vi "instance count allowed.vi"(8 "error in":errorcluster, 11 "WaveformAcq configuration in":refnum<class "WaveformAcq configuration.lvclass">) -> (0 "error out":errorcluster, 2 "instances allowed":i32, 3 "WaveformAcq configuration out":refnum<class "WaveformAcq configuration.lvclass">)   [LabVIEW 2017, in "WaveformAcq configuration.lvclass"]
uses:
  WaveformAcq configuration.lvclass
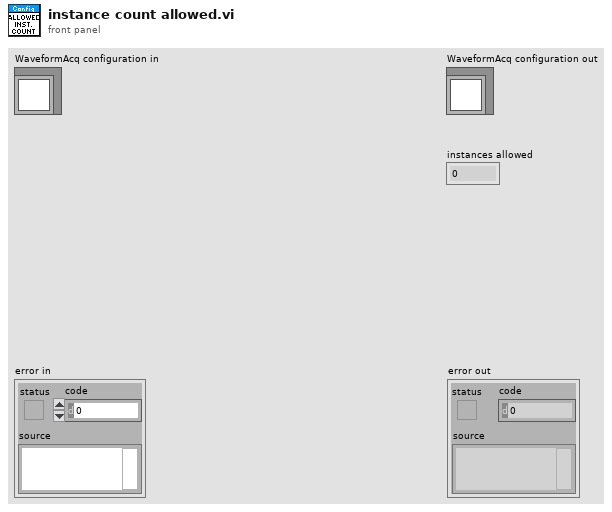
[diagram p1: front panel]
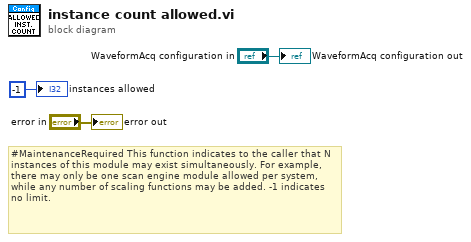
[diagram p0: block diagram]
diagram:
  # "#MaintenanceRequired This function indicates to the caller that N instances of this module may exist simultaneously. For example, there may only be one scan engine module allowed per system, while any number of scaling functions may be added. -1 indicates no limit."
  "error out" <- "error in"
  "WaveformAcq configuration out" <- "WaveformAcq configuration in"
  "instances allowed" <- -1 ("instances allowed")
